vi "[SubVI]EMGRMS.vi"(6 "Array 4":sgl[](array[numeric]), 7 "Array 2":sgl[](array[numeric]), 8 "Array 3":sgl[](array[numeric]), 9 "Number of samples (RMS)":i8, 10 "index":i32, 11 "Array":sgl[](array[numeric])) -> (0 "appended array":sgl[](array[numeric]))   [LabVIEW 2018]
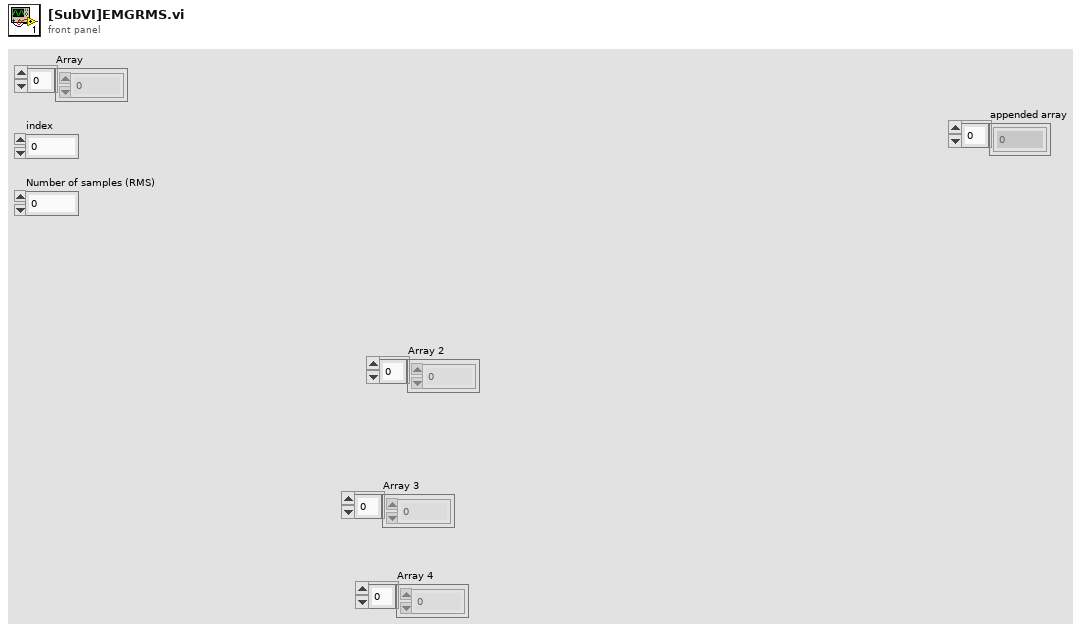
[diagram p1: front panel]
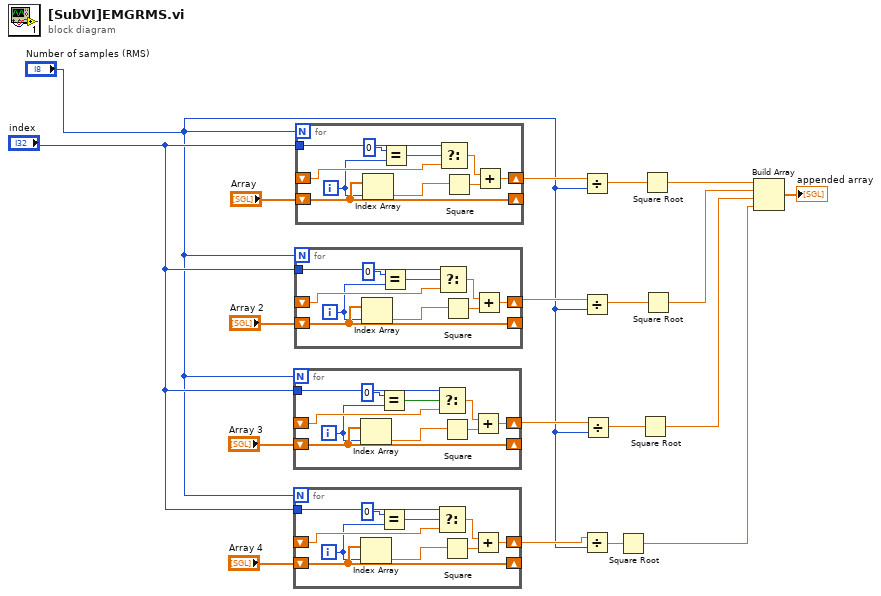
[diagram p0: block diagram]
diagram:
  n1 = for {
    N: "Number of samples (RMS)" -> [_]
    shift-right: [w28] -> w12
    shift-left: _ -> [w25]
    tunnel: "index" -> [w26]
    shift-right: [w22] -> _
    shift-left: "Array 3" -> [w22]
    i -> [w21]
    n2 = Index Array(array=w22, index=w21) -> (element=w23:sgl)
    n3 = Equal?(x=0 ("y"), y=w21) -> (x = y?=w27:bool)
    n4 = Select(t=w26, s=w27, f=w25) -> (s? t:f=w24:sgl)
    n5 = Square(x=w23) -> (x^2=w29:sgl)
    n6 = Add(x=w24, y=w29) -> (x+y=w28:sgl)
  }
  n7 = for {
    N: "Number of samples (RMS)" -> [_]
    shift-right: [w38] -> w13
    shift-left: _ -> [w35]
    tunnel: "index" -> [w36]
    shift-right: [w32] -> _
    shift-left: "Array 4" -> [w32]
    i -> [w31]
    n8 = Index Array(array=w32, index=w31) -> (element=w33:sgl)
    n9 = Equal?(x=0 ("y"), y=w31) -> (x = y?=w37:bool)
    n10 = Select(t=w36, s=w37, f=w35) -> (s? t:f=w34:sgl)
    n11 = Square(x=w33) -> (x^2=w39:sgl)
    n12 = Add(x=w34, y=w39) -> (x+y=w38:sgl)
  }
  n13 = for {
    N: "Number of samples (RMS)" -> [_]
    shift-right: [w48] -> w11
    shift-left: _ -> [w45]
    tunnel: "index" -> [w46]
    shift-right: [w42] -> _
    shift-left: "Array 2" -> [w42]
    i -> [w41]
    n14 = Index Array(array=w42, index=w41) -> (element=w43:sgl)
    n15 = Equal?(x=0 ("y"), y=w41) -> (x = y?=w47:bool)
    n16 = Select(t=w46, s=w47, f=w45) -> (s? t:f=w44:sgl)
    n17 = Square(x=w43) -> (x^2=w49:sgl)
    n18 = Add(x=w44, y=w49) -> (x+y=w48:sgl)
  }
  n19 = for {
    N: "Number of samples (RMS)" -> [_]
    shift-right: [w58] -> w14
    shift-left: _ -> [w55]
    tunnel: "index" -> [w56]
    shift-right: [w52] -> _
    shift-left: "Array" -> [w52]
    i -> [w51]
    n20 = Index Array(array=w52, index=w51) -> (element=w53:sgl)
    n21 = Equal?(x=0 ("y"), y=w51) -> (x = y?=w57:bool)
    n22 = Select(t=w56, s=w57, f=w55) -> (s? t:f=w54:sgl)
    n23 = Square(x=w53) -> (x^2=w59:sgl)
    n24 = Add(x=w54, y=w59) -> (x+y=w58:sgl)
  }
  n25 = Divide(x=w14, y="Number of samples (RMS)") -> (x/y=w2:sgl)
  n26 = Divide(x=w11, y="Number of samples (RMS)") -> (x/y=w4:sgl)
  n27 = Divide(x=w13, y="Number of samples (RMS)") -> (x/y=w8:sgl)
  n28 = Divide(x=w12, y="Number of samples (RMS)") -> (x/y=w6:sgl)
  n29 = Square Root(x=w8) -> (sqrt(x)=w7:sgl)
  n30 = Square Root(x=w6) -> (sqrt(x)=w5:sgl)
  n31 = Square Root(x=w2) -> (sqrt(x)=w1:sgl)
  n32 = Square Root(x=w4) -> (sqrt(x)=w3:sgl)
  n33 = Build Array(w1, w3, w5, w7) -> (→"appended array":sgl[])
